vi "ReloadChannelMonitoring.vi"(7 "LabVIEW Web Service Request":refnum<class "Web Request.lvclass">) -> ()   [LabVIEW 2018]
uses:
  <vilib>/wsapi/Web Request.lvclass
panel:
  in  "Channel":i32
  in  "error in (no error)":errorcluster
  # "Use the Web Service Request input terminal to call the VIs on the Web Services palette. Do not remove it from the connector pane unless you don't need access to the palette."
  # "Each additional control wired to the connector pane will be available as an input in the URL. To include an indicator in terminal-mode output (the default setting), it must also be wired to the connector pane."
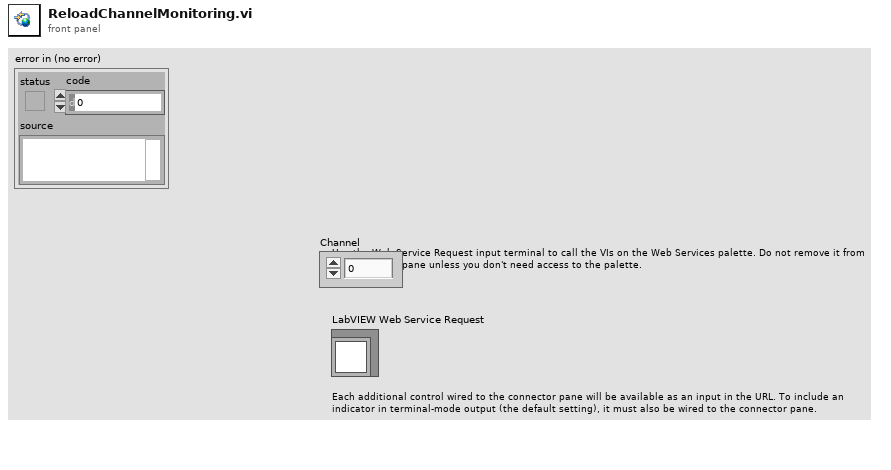
[diagram p1: front panel]
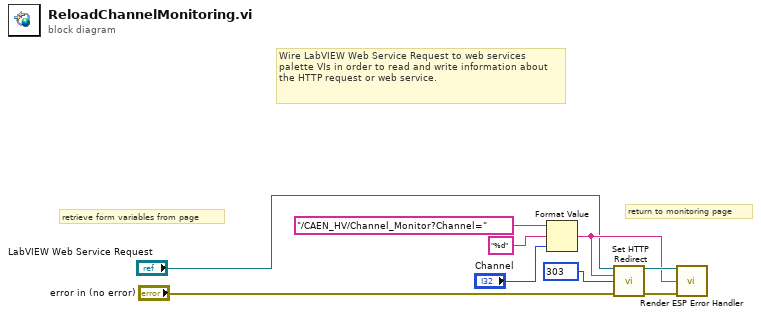
[diagram p0: block diagram]
diagram:
  w9 = 303 items=["100"=100, "101"=101, "200"=200, "201"=201, "202"=202, "203"=203, "204"=204, "205"=205, "206"=206, "300"=300, "301"=301, "302"=302, "303"=303, "304"=304, "305"=305, "306"=306, "307"=307, "400"=400, "401"=401, "402"=402, "403"=403, "404"=404, "405"=405, "406"=406, "407"=407, "408"=408, "409"=409, "410"=410, "411"=411, "412"=412, "413"=413, "414"=414, "415"=415, "416"=416, "417"=417, "500"=500, "501"=501, "502"=502, "503"=503, "504"=504, "505"=505] ("response code (307)")
  # "retrieve form variables from page"
  # "return to monitoring page"
  # "Wire LabVIEW Web Service Request to web services palette VIs in order to read and write information about the HTTP request or web service."
  n1 = Format Value(string ("")="/CAEN_HV/Channel_Monitor?Channel=" ("redirect URL"), format string="%d", value (0)="Channel") -> (output string=w4:string)
  n2 = call <vilib>:"Set HTTP Redirect.vi"("LabVIEW Web Service Request"="LabVIEW Web Service Request", "redirect URL"=w4, "response code (307)"=w9, "error in (no error)"="error in (no error)") -> ("LabVIEW Web Service Request out"=w7:refnum<class "Web Request.lvclass">, "error out"=w8:errorcluster)  [unwired: 10 in]
  n3 = call "Render ESP Error Handler.vi"("LabVIEW Web Service Request"=w7, "Link"=w4, "error in (no error)"=w8) -> ()  [unwired: 11 in, 2 out]
